vi "subDAQ_SetAO.vi"(7 "Analog value array":dbl[](array[numeric]) format="%0.2f", 8 "error in (no error)":errorcluster, 11 "Analog line array":tag[](array[tag])) -> (0 "error out":errorcluster)   [LabVIEW 2015]
uses:
  <vilib>/DAQmx/write.llb/DAQmx Write (Analog DBL 1Chan 1Samp).vi
  <vilib>/DAQmx/create/channels.llb/DAQmx Create Channel (AO-Voltage-Basic).vi
  <vilib>/DAQmx/miscellaneous.llb/DAQmx Fill In Error Info.vi
panel:
  # "Set Analog Output signal"
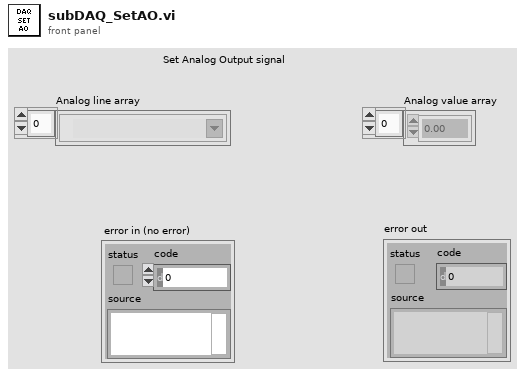
[diagram p1: front panel]
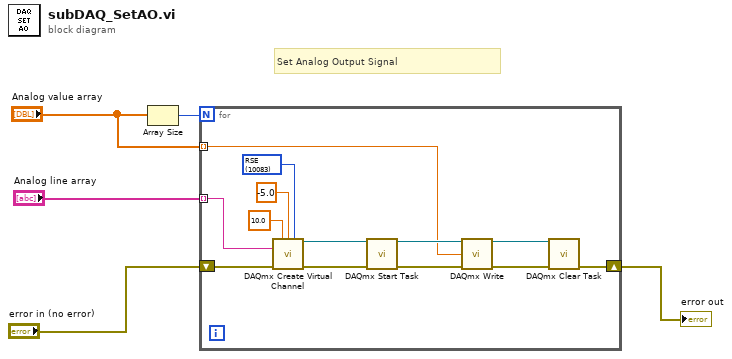
[diagram p0: block diagram]
diagram:
  # "Set Analog Output Signal"
  n1 = Array Size(array="Analog value array") -> (size(s)=w3:i32)
  n2 = for {
    N: w3 -> [_]
    shift-right: [w9] -> w4
    shift-left: "error in (no error)" -> [w10]
    tunnel: "Analog value array" -> [w8] mode=indexing
    tunnel: "Analog line array" -> [w7] mode=indexing
    w6 = 10083 items=["Default"=-1, "RSE"=10083, "Differential"=10106, "Pseudodifferential"=12529] ("output terminal configuration")
    n3 = call-poly <vilib>:"DAQmx Create Virtual Channel.vi"("maximum value"=10.0, "minimum value"=-5.0, "output terminal configuration"=w6, "physical channels"=w7, "error in"=w10) -> ("task out"=w13:refnum<k21>, "error out"=w14:errorcluster)  [unwired: 4 in, 5 out]
    n4 = call <vilib>:"DAQmx Start Task.vi"("task/channels in"=w13, "error in"=w14) -> ("task out"=w12:refnum<k21>, "error out"=w11:errorcluster)  [unwired: 12 out]
    n5 = call-poly <vilib>:"DAQmx Write.vi"("task/channels in"=w12, "data"=w8, "error in"=w11) -> ("task out"=w18:refnum<k21>, "error out"=w17:errorcluster)  [unwired: 1 in, 10 out]
    n6 = call <vilib>:"DAQmx Clear Task.vi"("task in"=w18, "error in"=w17) -> ("error out"=w9:errorcluster)  [unwired: 13 out]
  }
  "error out" <- w4
